vi "Pre Launch Init.vi"(11 "AE75TX in":refnum<class "AE75TX.lvclass">) -> (0 "error out":errorcluster, 3 "AE75TX out":refnum<class "AE75TX.lvclass">)   [LabVIEW 2018, in "AE75TX Actor.lvlib" / "AE75TX.lvclass"]
doc: "(<B>Filename</B>: Actor Framework.lvlib:Actor.lvclass:Pre Launch Init.vi)\n\nDefines behavior that occurs after the Launch Nested Actor method is invoked but before the actor's Actor Core method begins running.\n\nBy default, this method does nothing. A descendant class may override it to define behavior."
uses:
  AE75TX.lvclass
  AE75TX.lvclass/AE75TX.ctl
  <vilib>/ActorFramework/Actor/Actor.lvclass
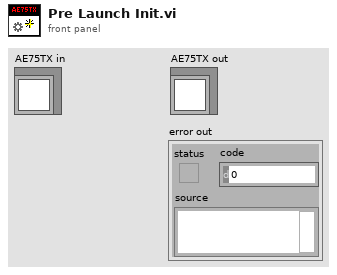
[diagram p1: front panel]
types:
  T1 = typedef "AE75TX Actor.lvlib/AE75TX.lvclass/AE75TX Notifiers.ctl" = cluster{"stop":refnum<notifier>}
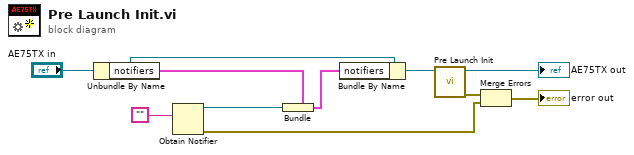
[diagram p0: block diagram]
diagram:
  n1 = Unbundle By Name("AE75TX in") -> ("notifiers"=w3:T1)
  n2 = Obtain Notifier(notification data type="") -> (notifier out=w4:refnum<notifier>, error out=w1:errorcluster)  [unwired: 3 in, 1 out]
  n3 = Bundle(cluster=w3, "stop"=w4) -> (w2:T1)
  n4 = Bundle By Name(cluster="AE75TX in", "notifiers"=w2) -> (w8:refnum<class "AE75TX.lvclass">)
  n5 = call-parent "Pre Launch Init.vi"("Actor in"=w8) -> ("error out"=w10:errorcluster, "Actor out"=→"AE75TX out":refnum<class "AE75TX.lvclass">)  [unwired: 9 in]
  n6 = Merge Errors(w10, w1) -> (→"error out":errorcluster)
